vi "Memory.Pointer.Error Info.vi"(11 "error (no error)":T1) -> (3 "error info":cluster{"code":i32, "description":string})   [LabVIEW 2016, in "Memory Manager.lvlib" / "Memory.Pointer.lvclass"]
uses:
  Memory.Pointer.lvclass
  Pointer.Void/Typedefs/Memory.Pointer.Errors.ctl
  Pointer.Void/Memory.Pointer.Void.lvclass
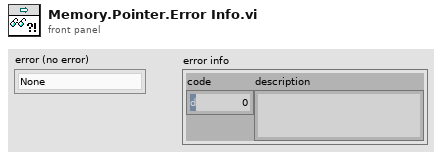
[diagram p1: front panel]
types:
  T1 = typedef "Memory Manager.lvlib/Memory.Pointer.Void.lvclass/Memory.Pointer.Errors.ctl" = enum16{"None", "Out of Range"}
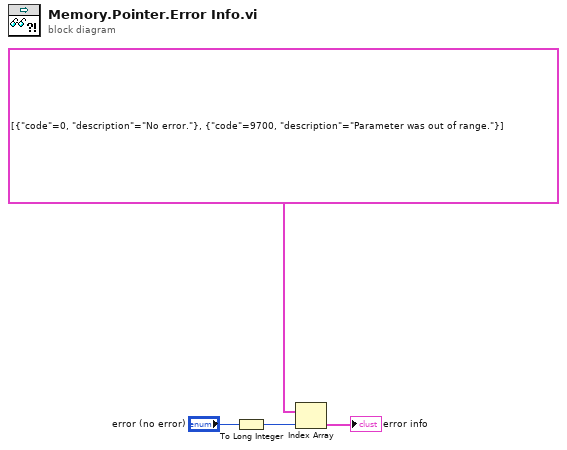
[diagram p0: block diagram]
diagram:
  n1 = To Long Integer(number="error (no error)") -> (32bit integer=w3:i32)
  n2 = Index Array(array=cluster{"code":i32, "description":string}[] [{"code"=0, "description"="No error."}, {"code"=9700, "description"="Parameter was out of range."}] ("error info"), index=w3) -> (element=→"error info":cluster{"code":i32, "description":string})
